vi "updateEngineeringList.vi"(8 "error in (no error)":errorcluster, 11 "ILCCommunications in":refnum<class "ILCCommunications.lvclass">) -> (0 "error out":errorcluster, 3 "ILCCommunications out":refnum<class "ILCCommunications.lvclass">)   [LabVIEW 2016, in "ILCCommunications.lvclass"]
uses:
  ILCCommunications.lvclass
  ILCCommunications.lvclass/ILCCommunications.ctl
  Common_RT_Modbus/ModbusBuffer/ModbusBuffer.lvclass/ModbusBuffer.ctl
  Common_RT_ILC/ILC/ILC.lvclass/ILC.ctl
  Common_RT_FAILC/FAILC/FAILC.lvclass/FAILC.ctl
  Common_RT_HPILC/HPILC/HPILC.lvclass/HPILC.ctl
  Common_RT_FAILC/FAILC/startBroadcastSetForceFrame.vi
  Common_RT_ILC/ILC/getILCData.vi
  Common_RT_FAILC/FAILC/populateBroadcastSetForceFrame.vi
  Common_RT_FAILC/FAILC/completeBroadcastSetForceFrame.vi
  Common_RT_HPILC/HPILC/startBroadcastStepMotorFrame.vi
  Common_RT_HPILC/HPILC/populateBroadcastStepMotorFrame.vi
  Common_RT_HPILC/HPILC/completeBroadcastStepMotorFrame.vi
  Common_RT_Modbus/ModbusBuffer/writeHeader.vi
  Common_RT_Modbus/ModbusBuffer/writeU8.vi
  Common_RT_FAILC/FAILC/determineSlewFlagValue.vi
  Common_RT_Modbus/ModbusBuffer/getIndex.vi
  Common_RT_Modbus/ModbusBuffer/writeI24.vi
  Common_RT_Modbus/ModbusBuffer/writeCRC.vi
  Common_RT_Modbus/ModbusBuffer/writeDelay.vi
  Common_RT_Modbus/ModbusBuffer/writeEndOfFrame.vi
  Common_RT_Modbus/ModbusBuffer/writeI8.vi
  Common_RT_Modbus/ModbusBuffer/writeByteInstruction.vi
  Common_RT_Modbus/ModbusBuffer/calculateCRC.vi
  Common_RT_FAILC/FAILC/FAILC.lvclass
  D:/Code/ts_M1M3Support/Common_RT_ILC/ILC/ILC.lvclass
  Common_RT_HPILC/HPILC/HPILC.lvclass
  Common_RT_Modbus/ModbusBuffer/ModbusBuffer.lvclass
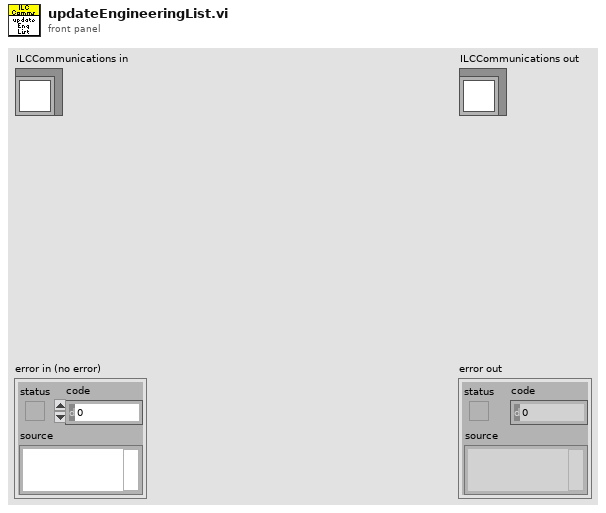
[diagram p1: front panel]
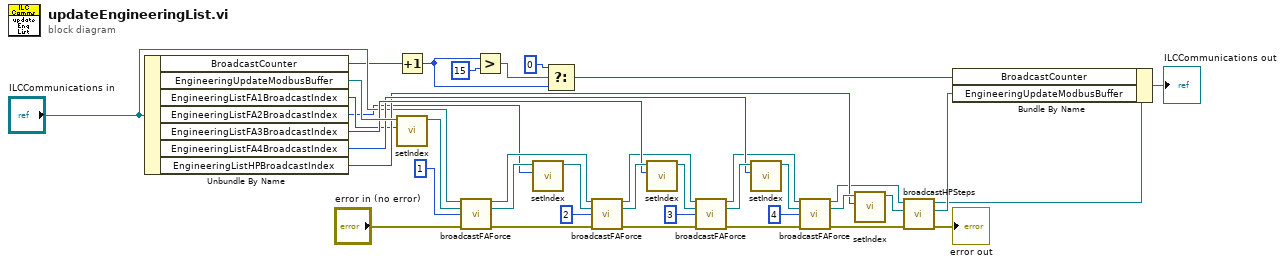
[diagram p0: block diagram]
diagram:
  n1 = Unbundle By Name("ILCCommunications in") -> ("BroadcastCounter"=w6:u8, "EngineeringUpdateModbusBuffer"=w35:refnum<class "ModbusBuffer.lvclass">, "EngineeringListFA1BroadcastIndex"=w5:i32, "EngineeringListFA2BroadcastIndex"=w4:i32, "EngineeringListFA3BroadcastIndex"=w25:i32, "EngineeringListFA4BroadcastIndex"=w24:i32, "EngineeringListHPBroadcastIndex"=w23:i32)
  n2 = Increment(x=w6) -> (x+1=w37:u8)
  n3 = call "setIndex.vi"("Index"=w5, "ModbusBuffer in"=w35) -> ("ModbusBuffer out"=w34:refnum<class "ModbusBuffer.lvclass">)  [unwired: 9 in]
  n4 = call "broadcastFAForce.vi"("ILCCommunications in"="ILCCommunications in", "ModbusBuffer in"=w34, "Subnet"=u8 1, "error in (no error)"="error in (no error)") -> ("ILCCommunications out"=w15:refnum<class "ILCCommunications.lvclass">, "ModbusBuffer out"=w33:refnum<class "ModbusBuffer.lvclass">, "error out"=w12:errorcluster)  [unwired: 9 in]
  n5 = Greater?(x=w37, y=u8 15) -> (0:w38:bool)
  n6 = call "setIndex.vi"("Index"=w4, "ModbusBuffer in"=w33) -> ("ModbusBuffer out"=w32:refnum<class "ModbusBuffer.lvclass">)  [unwired: 9 in]
  n7 = Select(t=u8 0, s=w38, f=w37) -> (s? t:f=w7:u8)
  n8 = call "broadcastFAForce.vi"("ILCCommunications in"=w15, "ModbusBuffer in"=w32, "Subnet"=u8 2, "error in (no error)"=w12) -> ("ILCCommunications out"=w16:refnum<class "ILCCommunications.lvclass">, "ModbusBuffer out"=w31:refnum<class "ModbusBuffer.lvclass">, "error out"=w11:errorcluster)  [unwired: 9 in]
  n9 = call "setIndex.vi"("Index"=w25, "ModbusBuffer in"=w31) -> ("ModbusBuffer out"=w30:refnum<class "ModbusBuffer.lvclass">)  [unwired: 9 in]
  n10 = call "broadcastFAForce.vi"("ILCCommunications in"=w16, "ModbusBuffer in"=w30, "Subnet"=u8 3, "error in (no error)"=w11) -> ("ILCCommunications out"=w17:refnum<class "ILCCommunications.lvclass">, "ModbusBuffer out"=w29:refnum<class "ModbusBuffer.lvclass">, "error out"=w10:errorcluster)  [unwired: 9 in]
  n11 = call "setIndex.vi"("Index"=w24, "ModbusBuffer in"=w29) -> ("ModbusBuffer out"=w28:refnum<class "ModbusBuffer.lvclass">)  [unwired: 9 in]
  n12 = call "broadcastFAForce.vi"("ILCCommunications in"=w17, "ModbusBuffer in"=w28, "Subnet"=u8 4, "error in (no error)"=w10) -> ("ILCCommunications out"=w18:refnum<class "ILCCommunications.lvclass">, "ModbusBuffer out"=w27:refnum<class "ModbusBuffer.lvclass">, "error out"=w9:errorcluster)  [unwired: 9 in]
  n13 = call "setIndex.vi"("Index"=w23, "ModbusBuffer in"=w27) -> ("ModbusBuffer out"=w26:refnum<class "ModbusBuffer.lvclass">)  [unwired: 9 in]
  n14 = call "broadcastHPSteps.vi"("error in (no error)"=w9, "ModbusBuffer in"=w26, "ILCCommunications in"=w18) -> ("error out"=→"error out":errorcluster, "ModbusBuffer out"=w3:refnum<class "ModbusBuffer.lvclass">, "ILCCommunications out"=w2:refnum<class "ILCCommunications.lvclass">)  [unwired: 6 in]
  n15 = Bundle By Name(cluster=w2, "BroadcastCounter"=w7, "EngineeringUpdateModbusBuffer"=w3) -> (→"ILCCommunications out":refnum<class "ILCCommunications.lvclass">)
